vi "HTTP.Dictionary to Header String.vi"(10 "Dictionary":variant) -> (2 "HTTP Header":string)   [LabVIEW 2013, in "Connection.WS_GOSPL.lvlib" / "Connection.WS.lvclass"]
uses:
  Connection.WS.lvclass
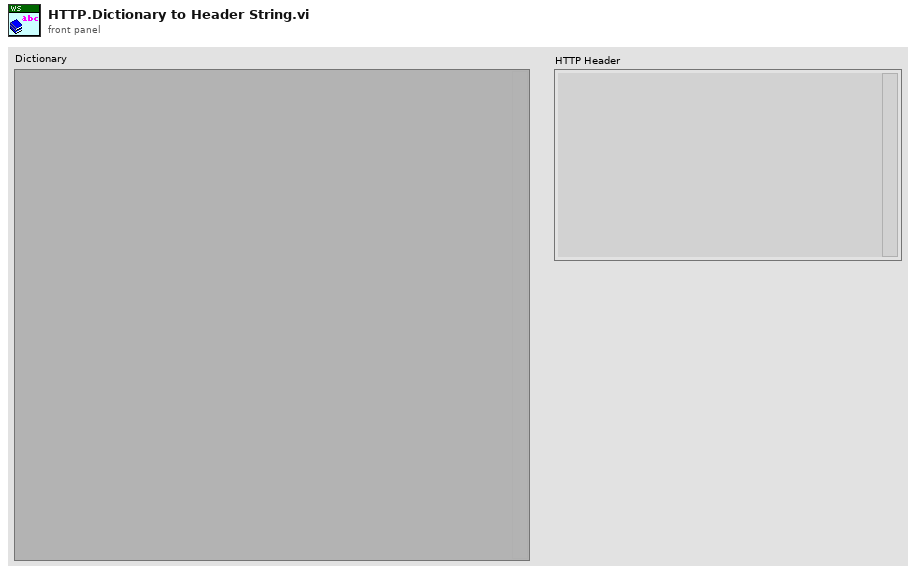
[diagram p1: front panel]
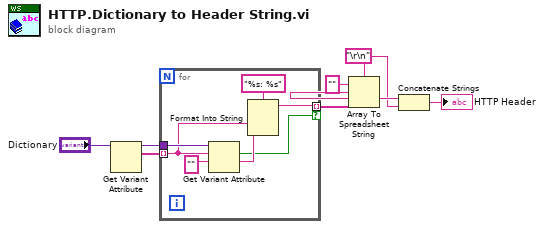
[diagram p0: block diagram]
diagram:
  w3 = "\r\n"
  n1 = Get Variant Attribute(Variant="Dictionary") -> (duplicate Variant=w8:variant, names=w7:string[])  [unwired: 3 in, 2 out]
  n2 = for {
    tunnel: w8 -> [w15]
    tunnel: w7 -> [w13] mode=indexing
    tunnel: [w10] -> w6 mode=indexing if=w9
    n3 = Get Variant Attribute(Variant=w15, name=w13, default value (empty Variant)="" ("format string")) -> (found=w9:bool, value=w12:string)  [unwired: 1 in, 2 out]
    n4 = Format Into String(format string="%s: %s", w13, w12) -> (resulting string=w10:string)  [unwired: 2 in, 1 out]
  }
  n5 = Array To Spreadsheet String(delimiter (Tab)=w3, array=w6, 3:"" ("format string")) -> (spreadsheet string=w4:string)
  n6 = Concatenate Strings(w4, w3) -> (→"HTTP Header":string)
